vi "DownloadPackageFromFTP.vi"(8 "error in (no error)":errorcluster, 10 "RemoteDirectory":string="/csm-vsc-extension", 11 "ftp":T1={"address"="vipm.nevstop.top", "remote port (21)"=1986, "userName"="anonymous", "passWord"="anonymous"}) -> (0 "error out":errorcluster, 2 "candidates":T2[](array[typedef])=[{"Name"="/Communicable-State-Machine/main/nevstop_lib_communicable_state_machine-2026.7.13.213856.vip", "Modify Timestamp"=timestamp(3866767278 s since 1904-01-01), "Dir-File Type"=enum."File", "Unique Id"="", "Permissions"="r", "Unix Mode"=0, "Owner"="", "Group"="14835828", "FileSize"=0}, {"Name"="/Communicable-State-Machine/Dev_2026Q2/nevstop_lib_communicable_state_machine-2026.7.13.161203.vip", "Modify Timestamp"=timestamp(3866747666 s since 1904-01-01), "Dir-File Type"=enum."File", "Unique Id"="", "Permissions"="r", "Unix Mode"=0, "Owner"="", "Group"="14835819", "FileSize"=0}, {"Name"="/Communicable-State-Machine/Dev_2026Q2/nevstop_lib_communicable_state_machine-2026.7.13.144427.vip", "Modify Timestamp"=timestamp(3866742430 s since 1904-01-01), "Dir-File Type"=enum."File", "Unique Id"="", "Permissions"="r", "Unix Mode"=0, "Owner"="", "Group"="14835826", "FileSize"=0}, {"Name"="/Communicable-State-Machine/Dev_2026Q2/nevstop_lib_communicable_state_machine-2026.6.23.213710.vip", "Modify Timestamp"=timestamp(3865039247 s since 1904-01-01), "Dir-File Type"=enum."File", "Unique Id"="", "Permissions"="r", "Unix Mode"=0, "Owner"="", "Group"="14835659", "FileSize"=0}, {"Name"="/Communicable-State-Machine/Dev_2026Q2/nevstop_lib_communicable_state_machine-2026.6.8.165946.vip", "Modify Timestamp"=timestamp(3863726720 s since 1904-01-01), "Dir-File Type"=enum."File", "Unique Id"="", "Permissions"="r", "Unix Mode"=0, "Owner"="", "Group"="14835575", "FileSize"=0}, {"Name"="/Communicable-State-Machine/Dev_2026Q2/nevstop_lib_communicable_state_machine-2026.6.4.94912.vip", "Modify Timestamp"=timestamp(3863355172 s since 1904-01-01), "Dir-File Type"=enum."File", "Unique Id"="", "Permissions"="r", "Unix Mode"=0, "Owner"="", "Group"="14835578", "FileSize"=0}, {"Name"="/Communicable-State-Machine/Dev_2026Q2/nevstop_lib_communicable_state_machine-2026.6.3.144755.vip", "Modify Timestamp"=timestamp(3863286682 s since 1904-01-01), "Dir-File Type"=enum."File", "Unique Id"="", "Permissions"="r", "Unix Mode"=0, "Owner"="", "Group"="14835537", "FileSize"=0}, {"Name"="/Communicable-State-Machine/Dev_2026Q2/nevstop_lib_communicable_state_machine-2026.5.9.214819.vip", "Modify Timestamp"=timestamp(3861151816 s since 1904-01-01), "Dir-File Type"=enum."File", "Unique Id"="", "Permissions"="r", "Unix Mode"=0, "Owner"="", "Group"="14832989", "FileSize"=0}, {"Name"="/Communicable-State-Machine/Dev_2026Q2/nevstop_lib_communicable_state_machine-2026.5.9.212614.vip", "Modify Timestamp"=timestamp(3861150433 s since 1904-01-01), "Dir-File Type"=enum."File", "Unique Id"="", "Permissions"="r", "Unix Mode"=0, "Owner"="", "Group"="14832830", "FileSize"=0}, {"Name"="/Communicable-State-Machine/Dev_2026Q2/nevstop_lib_communicable_state_machine-2026.5.9.203418.vip", "Modify Timestamp"=timestamp(3861147324 s since 1904-01-01), "Dir-File Type"=enum."File", "Unique Id"="", "Permissions"="r", "Unix Mode"=0, "Owner"="", "Group"="14832881", "FileSize"=0}, {"Name"="/Communicable-State-Machine/Dev_2026Q2/nevstop_lib_communicable_state_machine-2026.5.7.133148.vip", "Modify Timestamp"=timestamp(3860949194 s since 1904-01-01), "Dir-File Type"=enum."File", "Unique Id"="", "Permissions"="r", "Unix Mode"=0, "Owner"="", "Group"="14831281", "FileSize"=0}, {"Name"="/Communicable-State-Machine/Dev_2026Q2/nevstop_lib_communicable_state_machine-2026.5.7.110424.vip", "Modify Timestamp"=timestamp(3860940304 s since 1904-01-01), "Dir-File Type"=enum."File", "Unique Id"="", "Permissions"="r", "Unix Mode"=0, "Owner"="", "Group"="14829584", "FileSize"=0}, {"Name"="/Communicable-State-Machine/main/nevstop_lib_communicable_state_machine-2026.4.10.134916.vip", "Modify Timestamp"=timestamp(3858617442 s since 1904-01-01), "Dir-File Type"=enum."File", "Unique Id"="", "Permissions"="r", "Unix Mode"=0, "Owner"="", "Group"="14805816", "FileSize"=0}, {"Name"="/Communicable-State-Machine/Dev_2026Q1/nevstop_lib_communicable_state_machine-2026.4.10.132448.vip", "Modify Timestamp"=timestamp(3858615965 s since 1904-01-01), "Dir-File Type"=enum."File", "Unique Id"="", "Permissions"="r", "Unix Mode"=0, "Owner"="", "Group"="14805828", "FileSize"=0}, {"Name"="/Communicable-State-Machine/Dev_2026Q1/nevstop_lib_communicable_state_machine-2026.4.9.150129.vip", "Modify Timestamp"=timestamp(3858535689 s since 1904-01-01), "Dir-File Type"=enum."File", "Unique Id"="", "Permissions"="r", "Unix Mode"=0, "Owner"="", "Group"="14805636", "FileSize"=0}, {"Name"="/Communicable-State-Machine/Dev_2026Q1/nevstop_lib_communicable_state_machine-2026.4.8.203923.vip", "Modify Timestamp"=timestamp(3858469358 s since 1904-01-01), "Dir-File Type"=enum."File", "Unique Id"="", "Permissions"="r", "Unix Mode"=0, "Owner"="", "Group"="14805580", "FileSize"=0}, {"Name"="/Communicable-State-Machine/Dev_2026Q1/nevstop_lib_communicable_state_machine-2026.4.8.163515.vip", "Modify Timestamp"=timestamp(3858455036 s since 1904-01-01), "Dir-File Type"=enum."File", "Unique Id"="", "Permissions"="r", "Unix Mode"=0, "Owner"="", "Group"="14824281", "FileSize"=0}, {"Name"="/Communicable-State-Machine/Dev_2026Q1/nevstop_lib_communicable_state_machine-2026.3.6.173645.vip", "Modify Timestamp"=timestamp(3855607435 s since 1904-01-01), "Dir-File Type"=enum."File", "Unique Id"="", "Permissions"="r", "Unix Mode"=0, "Owner"="", "Group"="14688079", "FileSize"=0}, {"Name"="/Communicable-State-Machine/Dev_2026Q1/nevstop_lib_communicable_state_machine-2026.3.6.163725.vip", "Modify Timestamp"=timestamp(3855603885 s since 1904-01-01), "Dir-File Type"=enum."File", "Unique Id"="", "Permissions"="r", "Unix Mode"=0, "Owner"="", "Group"="14690118", "FileSize"=0}, {"Name"="/Communicable-State-Machine/Dev_2026Q1/nevstop_lib_communicable_state_machine-2026.3.6.153325.vip", "Modify Timestamp"=timestamp(3855600077 s since 1904-01-01), "Dir-File Type"=enum."File", "Unique Id"="", "Permissions"="r", "Unix Mode"=0, "Owner"="", "Group"="14690078", "FileSize"=0}, {"Name"="/Communicable-State-Machine/Dev_2026Q1/nevstop_lib_communicable_state_machine-2026.3.6.143002.vip", "Modify Timestamp"=timestamp(3855596263 s since 1904-01-01), "Dir-File Type"=enum."File", "Unique Id"="", "Permissions"="r", "Unix Mode"=0, "Owner"="", "Group"="14709368", "FileSize"=0}, {"Name"="/Communicable-State-Machine/Dev_2026Q1/nevstop_lib_communicable_state_machine-2026.2.13.135900.vip", "Modify Timestamp"=timestamp(3853779988 s since 1904-01-01), "Dir-File Type"=enum."File", "Unique Id"="", "Permissions"="r", "Unix Mode"=0, "Owner"="", "Group"="14708144", "FileSize"=0}, {"Name"="/Communicable-State-Machine/Dev_2026Q1/nevstop_lib_communicable_state_machine-2026.2.10.103437.vip", "Modify Timestamp"=timestamp(3853508465 s since 1904-01-01), "Dir-File Type"=enum."File", "Unique Id"="", "Permissions"="r", "Unix Mode"=0, "Owner"="", "Group"="14699450", "FileSize"=0}, {"Name"="/Communicable-State-Machine/Dev_2026Q1/nevstop_lib_communicable_state_machine-2026.2.9.232846.vip", "Modify Timestamp"=timestamp(3853468522 s since 1904-01-01), "Dir-File Type"=enum."File", "Unique Id"="", "Permissions"="r", "Unix Mode"=0, "Owner"="", "Group"="14697532", "FileSize"=0}, {"Name"="/Communicable-State-Machine/Dev_2026Q1/nevstop_lib_communicable_state_machine-2026.2.9.181822.vip", "Modify Timestamp"=timestamp(3853449832 s since 1904-01-01), "Dir-File Type"=enum."File", "Unique Id"="", "Permissions"="r", "Unix Mode"=0, "Owner"="", "Group"="14689701", "FileSize"=0}, {"Name"="/Communicable-State-Machine/Dev_2026Q1/nevstop_lib_communicable_state_machine-2026.2.9.174537.vip", "Modify Timestamp"=timestamp(3853447914 s since 1904-01-01), "Dir-File Type"=enum."File", "Unique Id"="", "Permissions"="r", "Unix Mode"=0, "Owner"="", "Group"="14693982", "FileSize"=0}, {"Name"="/Communicable-State-Machine/Dev_2026Q1/nevstop_lib_communicable_state_machine-2026.2.9.162121.vip", "Modify Timestamp"=timestamp(3853442786 s since 1904-01-01), "Dir-File Type"=enum."File", "Unique Id"="", "Permissions"="r", "Unix Mode"=0, "Owner"="", "Group"="14707279", "FileSize"=0}, {"Name"="/Communicable-State-Machine/v2025.Q4/nevstop_lib_communicable_state_machine-2026.1.26.120535.vip", "Modify Timestamp"=timestamp(3852217354 s since 1904-01-01), "Dir-File Type"=enum."File", "Unique Id"="", "Permissions"="r", "Unix Mode"=0, "Owner"="", "Group"="14770366", "FileSize"=0}], 3 "localdir":path=path "C:/Users/nevstop/AppData/Local/Temp/nevstop-lab/nevstop_lib_communicable_state_machine-2026.7.13.213856.vip", 4 "Array":string[](array[string])=["00002026000000070000001300213856", "00002026000000070000001300161203", "00002026000000070000001300144427", "00002026000000060000002300213710", "00002026000000060000000800165946", "00002026000000060000000400094912", "00002026000000060000000300144755", "00002026000000050000000900214819", "00002026000000050000000900212614", "00002026000000050000000900203418", "00002026000000050000000700133148", "00002026000000050000000700110424", "00002026000000040000001000134916", "00002026000000040000001000132448", "00002026000000040000000900150129", "00002026000000040000000800203923", "00002026000000040000000800163515", "00002026000000030000000600173645", "00002026000000030000000600163725", "00002026000000030000000600153325", "00002026000000030000000600143002", "00002026000000020000001300135900", "00002026000000020000001000103437", "00002026000000020000000900232846", "00002026000000020000000900181822", "00002026000000020000000900174537", "00002026000000020000000900162121", "00002026000000010000002600120535"])   [LabVIEW 2017, in "_Try Beta Version of CSMF.lvlib"]
uses:
  _Try Beta Version of CSMF.lvlib
  FTP/controls/Dir-File Info.ctl
  FTP/controls/Dir-File Type.ctl
  FTP/FTP.lvclass
  2061708c-d6dc-4f75-a668-a505e5e90b10.vi
  e182ef79-5db2-4bc9-9b19-535b120173da.vi
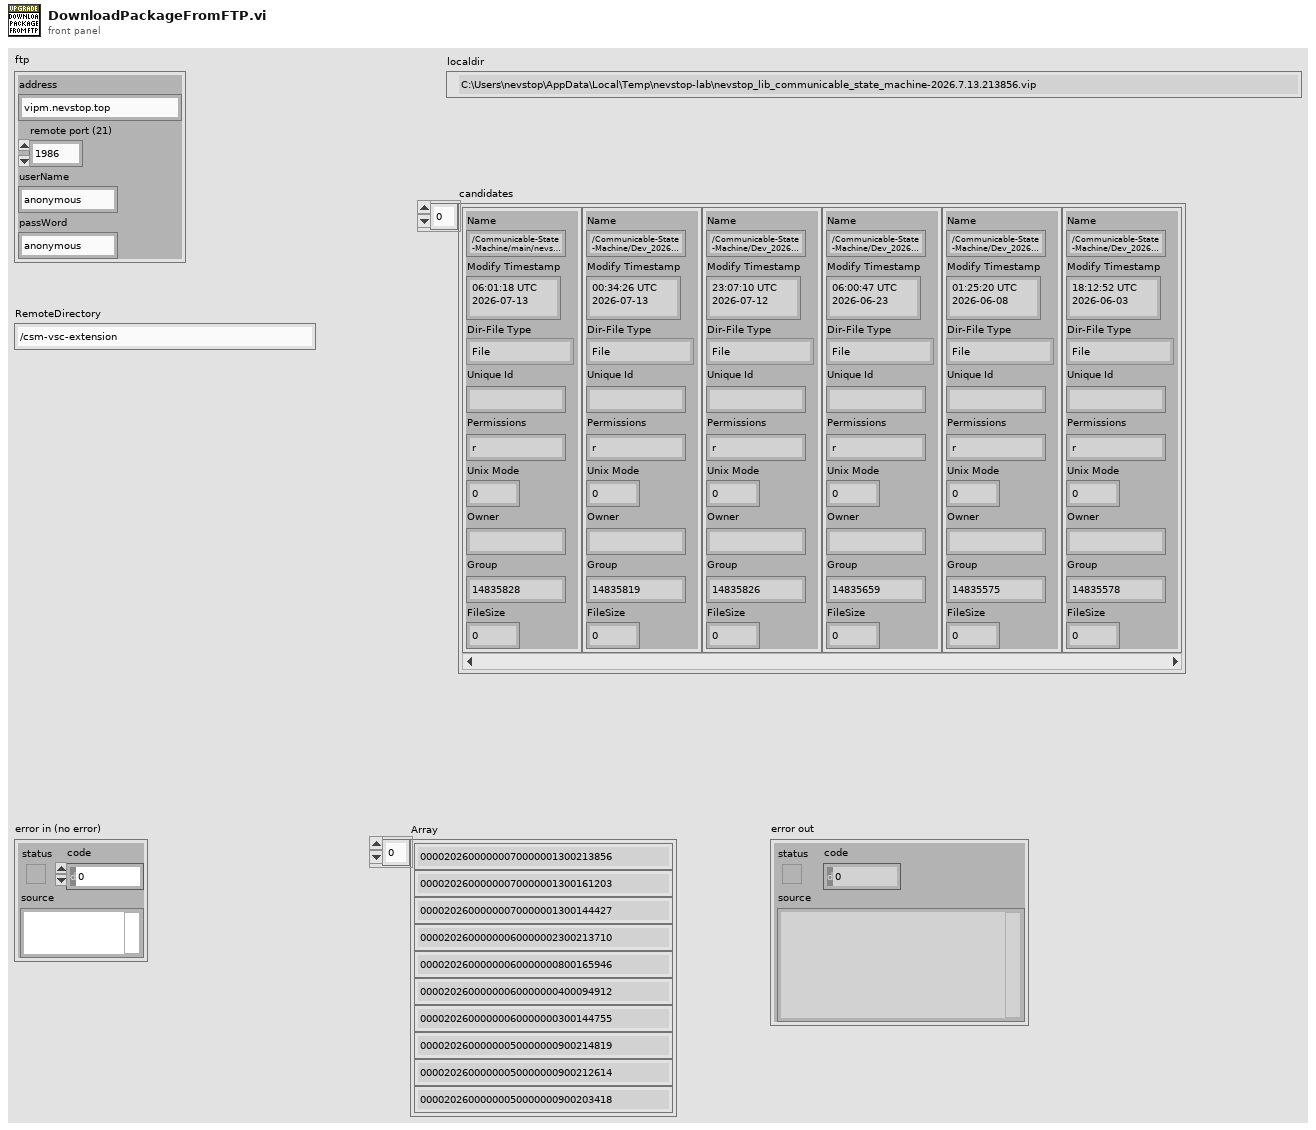
[diagram p1: front panel]
types:
  T1 = cluster{"address":string, "remote port (21)":u16, "userName":string, "passWord":string}
  T2 = typedef "FTP_UpgradeCSMF.lvlib/FTP.lvclass/Dir-File Info.ctl" = cluster{"Name":string, "Modify Timestamp":timestamp, "Dir-File Type":T3, "Unique Id":string, "Permissions":string, "Unix Mode":u16, "Owner":string, "Group":string, "FileSize":i64}
  T3 = typedef "FTP_UpgradeCSMF.lvlib/FTP.lvclass/Dir-File Type.ctl" = enum16{"File", "Listed Directory", "Parent Directory", "Directory", "Unknown"}
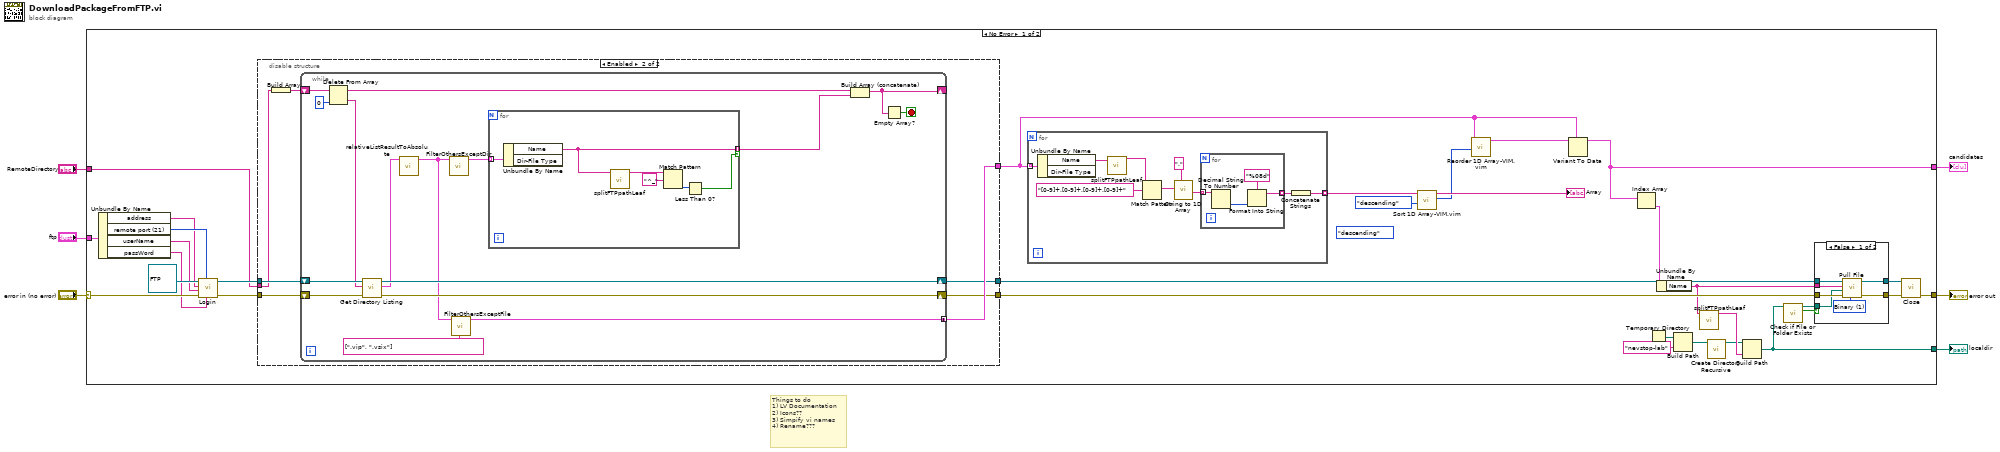
[diagram p0: block diagram]
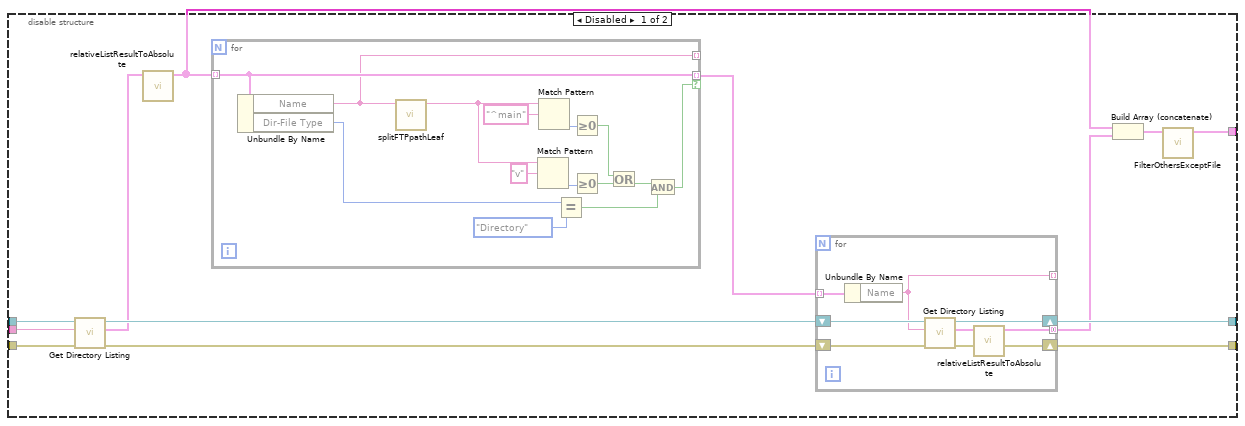
[diagram p3: hidden frame]
diagram:
  # "Things to do\n1) LV Documentation\n2) Icons??\n3) Simpify vi names\n4) Rename???"
  n1 = case shown="No Error" "error in (no error)" {
    selector: "error in (no error)" -> [w36 w125]
    tunnel: [w38 w125] -> w5
    tunnel: [w8 _] -> w4
    tunnel: [w18 _] -> w3
    tunnel: "ftp" -> [w16 _]
    tunnel: "RemoteDirectory" -> [w11 _]
    frame No Error {
      (unwired) enum16{"ascending", "descending"}."descending" ("Order")
      n2 = Unbundle By Name(w16) -> ("address"=w14:string, "remote port (21)"=w15:u16, "userName"=w13:string, "passWord"=w12:string)
      n3 = call "Login.vi"("passWord"=w12, "remote port (21)"=w15, "error in (no error)"=w36, "userName"=w13, "address"=w14, "FTP in"=refnum<class "FTP.lvclass"> refnum) -> ("error out"=w35:errorcluster, "FTP out"=w37:refnum<class "FTP.lvclass">)  [unwired: 4 in]
      n4 = disable-structure shown="Enabled" {
        disable-tunnel: w37 -> [w73 w102]
        disable-tunnel: w35 -> [w72 w101]
        disable-tunnel: [w68 w96] -> w34
        disable-tunnel: [w67 w97] -> w33
        disable-tunnel: [w62 w98] -> w28
        disable-tunnel: w11 -> [w61 w100]
        frame Disabled {
          n5 = call "Get Directory Listing.vi"("error in (no error)"=w72, "RemoteDirectory"=w61, "FTP in"=w73) -> ("error out"=w70:errorcluster, "Dir-File Info Array"=w64:T2[], "FTP out"=w71:refnum<class "FTP.lvclass">)  [unwired: 6 in]
          n6 = call "relativeListResultToAbsolute.vi"("Dir-File Info Array"=w64) -> ("Array"=w63:T2[])  [unwired: 10 in]
          n7 = for {
            tunnel: w63 -> [w89] mode=indexing
            tunnel: [w89] -> w69 mode=indexing if=w88
            tunnel: [w82] -> _ mode=indexing
            n8 = Unbundle By Name(w89) -> ("Name"=w82:string, "Dir-File Type"=w94:T3)
            n9 = call "splitFTPpathLeaf.vi"("Name"=w82) -> ("String"=w83:string)  [unwired: 10 in]
            n10 = Match Pattern(string=w83, regular expression="v") -> (offset past match=w92:i32)  [unwired: 1 in, 3 out]
            n11 = Match Pattern(string=w83, regular expression="^main") -> (offset past match=w87:i32)  [unwired: 1 in, 3 out]
            n12 = Equal?(x=w94, y=Dir-File_Type."Directory") -> (x = y?=w90:bool)
            n13 = Greater Or Equal To 0?(x=w87) -> (x >= 0?=w84:bool)
            n14 = Greater Or Equal To 0?(x=w92) -> (x >= 0?=w91:bool)
            n15 = Or(x=w84, y=w91) -> (x .or. y?=w85:bool)
            n16 = And(x=w85, y=w90) -> (x .and. y?=w88:bool)
          }
          n17 = for {
            tunnel: w69 -> [w79] mode=indexing
            tunnel: [w75] -> w66 mode=concatenating
            shift-right: [w77] -> w67
            shift-left: w71 -> [w81]
            shift-right: [w78] -> w68
            shift-left: w70 -> [w80]
            tunnel: [w74] -> _ mode=indexing
            n18 = Unbundle By Name(w79) -> ("Name"=w74:string)
            n19 = call "Get Directory Listing.vi"("error in (no error)"=w80, "RemoteDirectory"=w74, "FTP in"=w81) -> ("error out"=w78:errorcluster, "Dir-File Info Array"=w76:T2[], "FTP out"=w77:refnum<class "FTP.lvclass">)  [unwired: 6 in]
            n20 = call "relativeListResultToAbsolute.vi"("Dir-File Info Array"=w76) -> ("Array"=w75:T2[])  [unwired: 10 in]
          }
          n21 = Build Array (concatenate)(w63, w66) -> (w65:T2[])
          n22 = call "FilterOthersExceptFile.vi"("Array in"=w65) -> ("Array out"=w62:T2[])  [unwired: 10 in]
        }
        frame Enabled {
          n23 = Build Array(w100) -> (w99:string[])
          n24 = while {
            shift-right: [w116] -> w97
            shift-left: w102 -> [w118]
            shift-right: [w115] -> w96
            shift-left: w101 -> [w117]
            shift-right: [w106] -> _
            shift-left: w99 -> [w113]
            tunnel: [w110] -> w98 mode=concatenating
            stop <- w105 stop-if-true
            n25 = Delete From Array(array=w113, index=0) -> (deleted portion=w111:string, array with subset deleted=w107:string[])  [unwired: 1 in]
            n26 = call "Get Directory Listing.vi"("error in (no error)"=w117, "RemoteDirectory"=w111, "FTP in"=w118) -> ("error out"=w115:errorcluster, "Dir-File Info Array"=w114:T2[], "FTP out"=w116:refnum<class "FTP.lvclass">)  [unwired: 6 in]
            n27 = call "relativeListResultToAbsolute.vi"("Dir-File Info Array"=w114) -> ("Array"=w109:T2[])  [unwired: 10 in]
            n28 = call "FilterOthersExceptDir.vi"("Array in"=w109) -> ("Array out"=w108:T2[])  [unwired: 10 in]
            n29 = call "FilterOthersExceptFile.vi"("Extensions(.vip, .visx)"=string[] [".vip", ".vsix"], "Array in"=w109) -> ("Array out"=w110:T2[])  [unwired: 9 in]
            n30 = for {
              tunnel: w108 -> [w124] mode=indexing
              tunnel: [w123] -> w104 mode=indexing if=w119
              n31 = Unbundle By Name(w124) -> ("Name"=w123:string)  [unwired: 1 out]
              n32 = call "splitFTPpathLeaf.vi"("Name"=w123) -> ("String"=w120:string)  [unwired: 10 in]
              n33 = Match Pattern(string=w120, regular expression="^_") -> (offset past match=w121:i32)  [unwired: 1 in, 3 out]
              n34 = Less Than 0?(x=w121) -> (x < 0?=w119:bool)
            }
            n35 = Build Array (concatenate)(w107, w104) -> (w106:string[])
            n36 = Empty Array?(array=w106) -> (empty?=w105:bool)
          }
        }
      }
      n37 = for {
        tunnel: w28 -> [w56] mode=indexing
        tunnel: [w48] -> w32 mode=indexing
        n38 = Unbundle By Name(w56) -> ("Name"=w55:string)  [unwired: 1 out]
        n39 = call "splitFTPpathLeaf.vi"("Name"=w55) -> ("String"=w53:string)  [unwired: 10 in]
        n40 = Match Pattern(string=w53, regular expression="[0-9]+.[0-9]+.[0-9]+.[0-9]+") -> (match substring=w52:string)  [unwired: 1 in, 3 out]
        n41 = call "String to 1D Array.vi"("delimiter (Tab)"=".", "string"=w52) -> ("Array of Strings"=w50:string[])  [unwired: 9 in]
        n42 = for {
          tunnel: w50 -> [w60] mode=indexing
          tunnel: [w58] -> w49 mode=indexing
          n43 = Decimal String To Number(string=w60) -> (number=w57:i32)  [unwired: 2 in, 1 out]
          n44 = Format Into String(format string="%08d", w57) -> (resulting string=w58:string)  [unwired: 2 in, 1 out]
        }
        n45 = Concatenate Strings(w49) -> (w48:string)
      }
      n46 = call "Sort 1D Array-VIM.vim"("Order (ascending)"=enum16{"ascending", "descending"}."descending", "Array in"=w32) -> ("Sorted Pointers"=w30:i32[], "Sorted Array out"=→"Array":string[])  [unwired: 8 in]
      n47 = call "Reorder 1D Array-VIM.vim"("indices"=w30, "array"=w28) -> ("reordered array"=w29:T2[])  [unwired: 9 in]
      n48 = Variant To Data(type=w28, Variant=w29) -> (data=w18:T2[])  [unwired: 1 in, 1 out]
      n49 = Index Array(array=w18) -> (element=w25:T2)  [unwired: 1 in]
      n50 = Temporary Directory() -> (w24:path)
      n51 = Unbundle By Name(w25) -> ("Name"=w21:string)
      n52 = Build Path(base path=w24, name or relative path="nevstop-lab") -> (appended path=w23:path)
      n53 = call "splitFTPpathLeaf.vi"("Name"=w21) -> ("String"=w20:string)  [unwired: 10 in]
      n54 = call <vilib>:"Create Directory Recursive.vi"("directory"=w23) -> ("directory copy"=w19:path)  [unwired: 4 in, 2 out]
      n55 = Build Path(base path=w19, name or relative path=w20) -> (appended path=w8:path)
      n56 = call <vilib>:"Check if File or Folder Exists.vi"("path"=w8) -> ("file or folder exists?"=w9:bool, "dup path"=w10:path)  [unwired: 8 in, 1 out]
      n57 = case shown="False" w9 {
        tunnel: w34 -> [w44 w46]
        tunnel: w33 -> [w43 w47]
        tunnel: [w42 w47] -> w27
        tunnel: [w41 w46] -> w26
        tunnel: w21 -> [w40 _]
        tunnel: w10 -> [w39 _]
        frame False {
          w45 = u16 1 items=["ASCII", "Binary"] ("Type")
          n58 = call "Pull File.vi"("Type (Binary)"=w45, "error in (no error)"=w44, "Local FilePath"=w39, "FileName"=w40, "FTP in"=w43) -> ("error out"=w41:errorcluster, "FTP out"=w42:refnum<class "FTP.lvclass">)  [unwired: 5 in]
        }
        frame True {
        }
      }
      n59 = call "Close.vi"("error in (no error)"=w26, "FTP in"=w27) -> ("error out"=w38:errorcluster)  [unwired: 9 in]
    }
    frame Error {
    }
  }
  "error out" <- w5
  "localdir" <- w4
  "candidates" <- w3
